vi "LV SciSDK OSCILLOSCOPE DUAL RESET READ VALID FLAG.vi"(8 "error in (no error)":errorcluster, 9 "Oscilloscope Dual Handle In":T1) -> (0 "error out":errorcluster, 1 "Oscilloscope Dual Handle Out":T1)   [LabVIEW 2021]
uses:
  SciSDK_Labview.lvlib
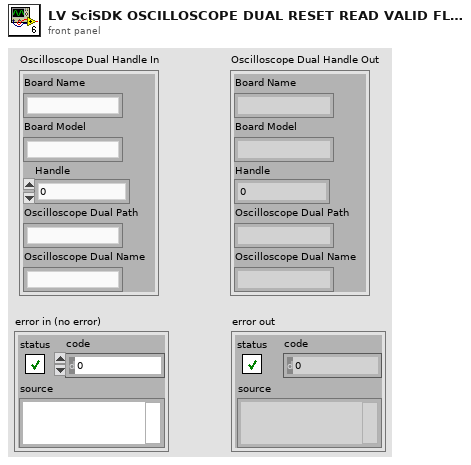
[diagram p1: front panel]
types:
  T1 = cluster{"Board Name":string, "Board Model":string, "Handle":u64, "Oscilloscope Dual Path":string, "Oscilloscope Dual Name":string}
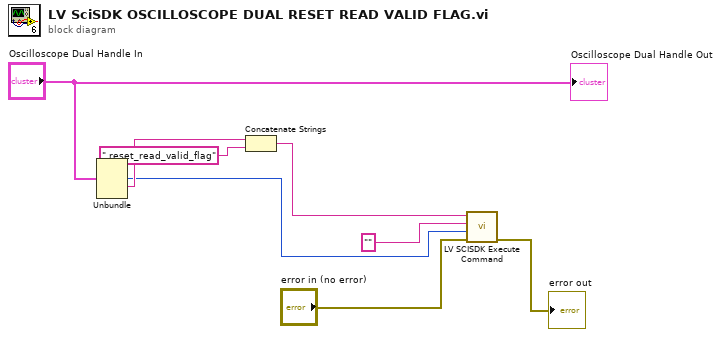
[diagram p0: block diagram]
diagram:
  n1 = Unbundle("Oscilloscope Dual Handle In") -> ("Handle"=w3:u64, "Oscilloscope Dual Path"=w7:string)  [unwired: 3 out]
  n2 = Concatenate Strings(w7, ".reset_read_valid_flag" ("string")) -> (w5:string)
  n3 = call "LV SCISDK Execute Command.vi"("error in (no error)"="error in (no error)", "handle"=w3, "value"="", "Path"=w5) -> ("error out"=→"error out":errorcluster)  [unwired: 5 in, 2 out]
  "Oscilloscope Dual Handle Out" <- "Oscilloscope Dual Handle In"
